vi "DevRef Data Base fg.vi"(9 "DevRef to Get":T11, 11 "Menu":T12) -> (0 "error out":errorcluster, 1 "Selected Sensor":T1, 2 "Selected Encoder":T4={"DevStatus"={"status"=FALSE, "code"=0, "source"=""}, "EncoderIndex"=enum."Invalid", "CounterIndex"=enum."Invalid", "DistancePerCount"=1.0, "Decoding Type"=enum."4x"}, 3 "Selected Solenoid":T8={"DevStatus"={"status"=FALSE, "code"=0, "source"=""}, "Solenoid Module"=enum."Solenoid Module 1", "Forward Solenoid Channel"=enum."Invalid", "Reverse Solenoid Channel"=enum."Invalid"}, 4 "autoshoot":T1, 5 "right drive encoder":T4={"DevStatus"={"status"=FALSE, "code"=0, "source"=""}, "EncoderIndex"=enum."Invalid", "CounterIndex"=enum."Invalid", "DistancePerCount"=1.0, "Decoding Type"=enum."4x"}, 6 "hotgoal":T1, 7 "left drive encoder":T4={"DevStatus"={"status"=FALSE, "code"=0, "source"=""}, "EncoderIndex"=enum."Invalid", "CounterIndex"=enum."Invalid", "DistancePerCount"=1.0, "Decoding Type"=enum."4x"}, 8 "2ball":T1)   [LabVIEW 2013]
uses:
  typedefs/fg_typedef.ctl
  typedefs/DevRef Type.ctl
  <vilib>/Rock Robotics/WPI/Solenoid/WPI_SolenoidDevRef.ctl
  <vilib>/Rock Robotics/SystemInterfaces/Typedef/FPGA_TypedefSolenoidModule.ctl
  <vilib>/Rock Robotics/WPI/Solenoid/WPI_SolenoidChannel.ctl
  <vilib>/Rock Robotics/WPI/DigitalInput/WPI_DigitalInputDevRef.ctl
  <vilib>/Rock Robotics/SystemInterfaces/DIO/FPGA_DIOChannel.ctl
  <vilib>/Rock Robotics/SystemInterfaces/Typedef/FPGA_TypedefDigitalModule.ctl
  <vilib>/Rock Robotics/WPI/Encoder/WPI_EncoderDevRef.ctl
  <vilib>/Rock Robotics/SystemInterfaces/Encoder/FPGA_EncoderIdx.ctl
  <vilib>/Rock Robotics/SystemInterfaces/Counter/FPGA_CounterCtrSystemIndex.ctl
  <vilib>/Rock Robotics/WPI/Encoder/WPI_EncoderType.ctl
panel:
  # "A Functional Global that stores refnums for \ncommonly used devices \nso as to not need to get them repeatedly"
  # "it is only set once"
  # "Option to Select Also..."
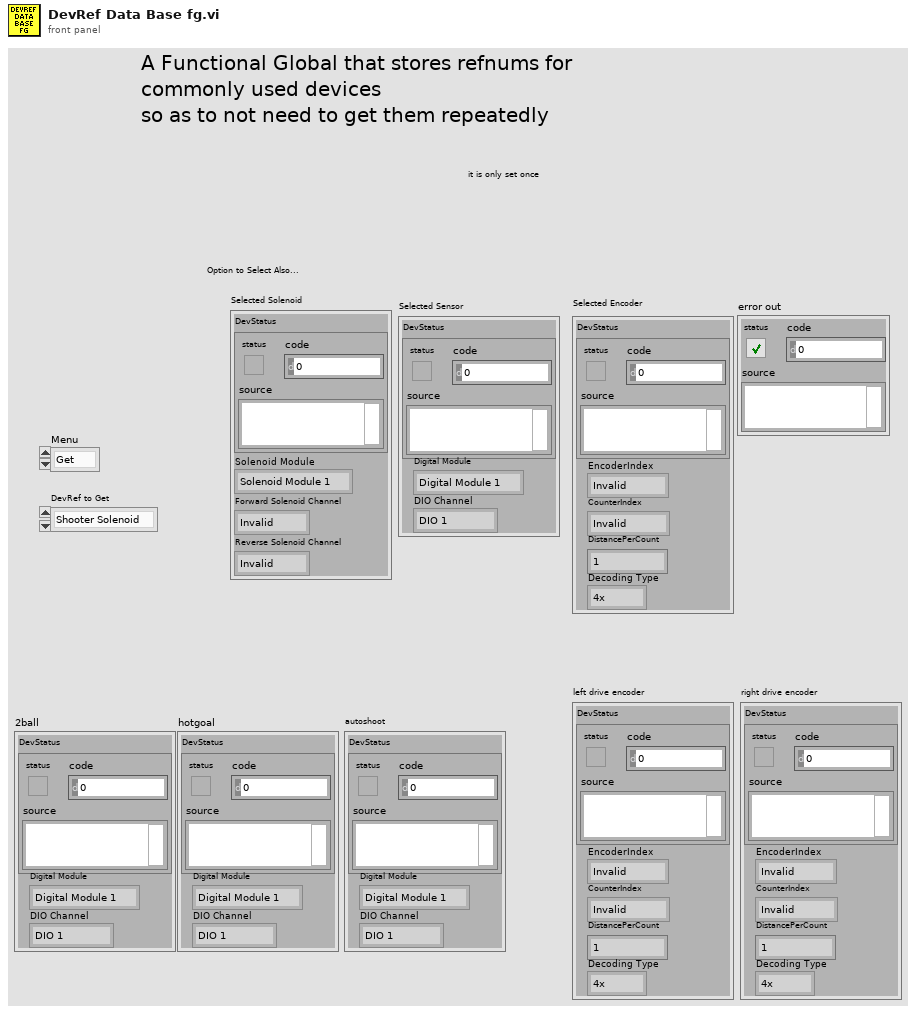
[diagram p1: front panel]
types:
  T1 = typedef "WPI_DigitalInputDevRef.ctl" = cluster{"DevStatus":errorcluster, "DIO Channel":T2, "Digital Module":T3}
  T2 = typedef "FPGA_DIOChannel.ctl" = enum8{"DIO 1", "DIO 2", "DIO 3", "DIO 4", "DIO 5", "DIO 6", "DIO 7", "DIO 8", "DIO 9", "DIO 10", "DIO 11", "DIO 12", "DIO 13", "DIO 14", "Invalid"}
  T3 = typedef "FPGA_TypedefDigitalModule.ctl" = enum16{"Digital Module 1", "Digital Module 2"}
  T4 = typedef "WPI_EncoderDevRef.ctl" = cluster{"DevStatus":errorcluster, "EncoderIndex":T5, "CounterIndex":T6, "DistancePerCount":dbl, "Decoding Type":T7}
  T5 = typedef "FPGA_EncoderIdx.ctl" = enum8{"Enc 0", "Enc 1", "Enc 2", "Enc 3", "Invalid"}
  T6 = typedef "FPGA_CounterCtrSystemIndex.ctl" = enum8{"Ctr 0", "Ctr 1", "Ctr 2", "Ctr 3", "Ctr 4", "Ctr 5", "Ctr 6", "Ctr 7", "Invalid"}
  T7 = typedef "WPI_EncoderType.ctl" = enum16{"1x", "2x", "4x"}
  T8 = typedef "WPI_SolenoidDevRef.ctl" = cluster{"DevStatus":errorcluster, "Solenoid Module":T9, "Forward Solenoid Channel":T10, "Reverse Solenoid Channel":T10}
  T9 = typedef "FPGA_TypedefSolenoidModule.ctl" = enum16{"Solenoid Module 1", "Solenoid Module 2"}
  T10 = typedef "WPI_SolenoidChannel.ctl" = enum8{"Solenoid 1", "Solenoid 2", "Solenoid 3", "Solenoid 4", "Solenoid 5", "Solenoid 6", "Solenoid 7", "Solenoid 8", "Invalid"}
  T11 = typedef "DevRef Type.ctl" = enum16{"Shooter Solenoid", "Latch Solenoid", "Right Up Sensor", "Right Down Sensor", "Hold Sensor", "Arm Encoder"}
  T12 = typedef "fg_typedef.ctl" = enum16{"Get", "Set"}
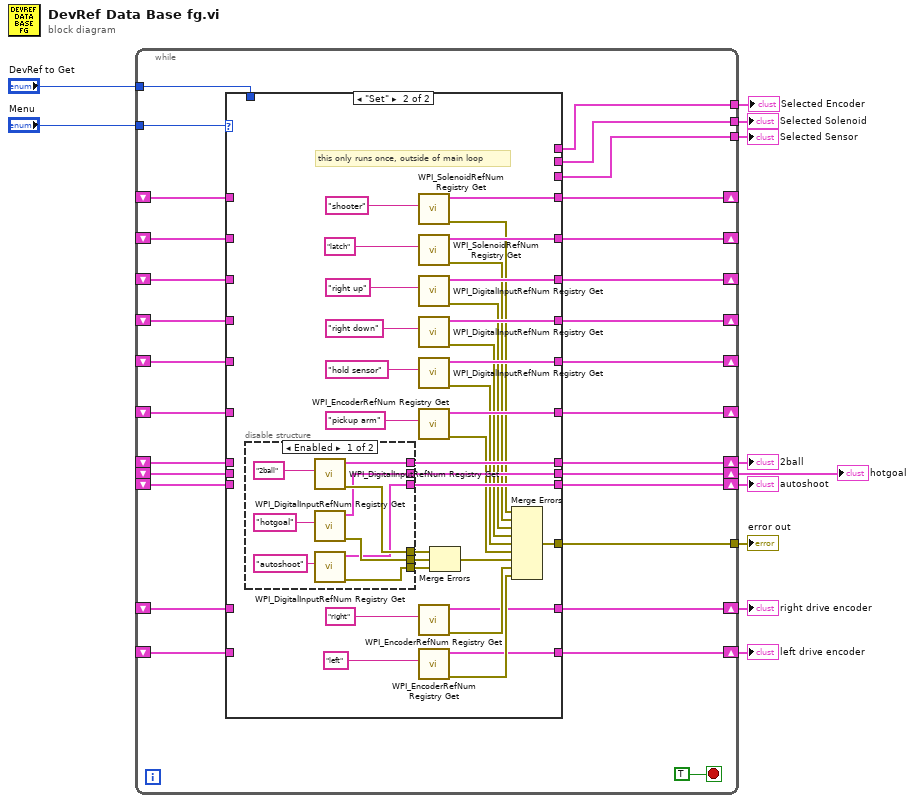
[diagram p0: block diagram]
diagram:
  n1 = while {
    shift-right: [w34] -> _
    shift-left: _ -> [w39]
    shift-right: [w33] -> _
    shift-left: _ -> [w38]
    shift-right: [w32] -> _
    shift-left: _ -> [w36]
    shift-right: [w31] -> _
    shift-left: _ -> [w35]
    tunnel: "Menu" -> [w37]
    shift-right: [w29] -> _
    shift-left: _ -> [w30]
    tunnel: "DevRef to Get" -> [w28]
    tunnel: [w27] -> w9
    tunnel: [w26] -> w8
    shift-right: [w24] -> _
    shift-left: _ -> [w25]
    tunnel: [w23] -> w7
    shift-right: [w22] -> w3
    shift-left: _ -> [w21]
    shift-right: [w20] -> w5
    shift-left: _ -> [w17]
    shift-right: [w19] -> w4
    shift-left: _ -> [w16]
    tunnel: [w18] -> w6
    shift-right: [w15] -> w2
    shift-left: _ -> [w13]
    shift-right: [w14] -> w1
    shift-left: _ -> [w12]
    stop <- TRUE stop-if-true
    n2 = case shown="\"Set\"" w37 {
      tunnel: w39 -> [w60 _]
      tunnel: w38 -> [w59 _]
      tunnel: w36 -> [w58 _]
      tunnel: w35 -> [w57 _]
      tunnel: [w49 w122] -> w34
      tunnel: [w50 w121] -> w33
      tunnel: [w51 w120] -> w32
      tunnel: [w52 w119] -> w31
      tunnel: w30 -> [w56 _]
      tunnel: [w53 w118] -> w29
      tunnel: w28 -> [w61 _]
      tunnel: [w55 _] -> w27
      tunnel: [w54 _] -> w26
      tunnel: w25 -> [w48 _]
      tunnel: [w47 w116] -> w24
      tunnel: [w46 _] -> w23
      tunnel: [w43 w115] -> w22
      tunnel: w21 -> [w43 _]
      tunnel: [w45 w104] -> w20
      tunnel: [w44 w103] -> w19
      tunnel: [_ w102] -> w18
      tunnel: w17 -> [w45 _]
      tunnel: w16 -> [w44 _]
      tunnel: [w42 w129] -> w15
      tunnel: [w41 w128] -> w14
      tunnel: w13 -> [w42 _]
      tunnel: w12 -> [w41 _]
      frame "Get", Default {
        # "always get the autobox"
        # "always get the drive encoders"
        n3 = case shown="\"Shooter Solenoid\", Default" w61 {
          tunnel: w60 -> [w63 w73 w79 w85 w91 w97]
          tunnel: w59 -> [w64 w72 w78 w84 w90 w96]
          tunnel: w58 -> [w65 w71 w77 w83 w89 w95]
          tunnel: w57 -> [w66 w70 w76 w82 w88 w94]
          tunnel: w56 -> [w67 w69 w75 w81 w87 w93]
          tunnel: [w63 w72 _ _ _ _] -> w55
          tunnel: [_ _ w77 w82 w87 _] -> w54
          tunnel: [w67 w69 w75 w81 w87 w93] -> w53
          tunnel: [w66 w70 w76 w82 w88 w94] -> w52
          tunnel: [w65 w71 w77 w83 w89 w95] -> w51
          tunnel: [w64 w72 w78 w84 w90 w96] -> w50
          tunnel: [w63 w73 w79 w85 w91 w97] -> w49
          tunnel: w48 -> [w62 w68 w74 w80 w86 w92]
          tunnel: [w62 w68 w74 w80 w86 w92] -> w47
          tunnel: [_ _ _ _ _ w92] -> w46
          frame "Shooter Solenoid", Default {
          }
          frame "Latch Solenoid" {
          }
          frame "Right Up Sensor" {
          }
          frame "Right Down Sensor" {
          }
          frame "Hold Sensor" {
          }
          frame "Arm Encoder" {
          }
        }
      }
      frame "Set" {
        # "this only runs once, outside of main loop"
        n4 = disable-structure shown="Enabled" {
          disable-tunnel: [w134 _] -> w115
          disable-tunnel: [w131 _] -> w129
          disable-tunnel: [w130 _] -> w128
          disable-tunnel: [w138 _] -> w101
          disable-tunnel: [w137 _] -> w100
          disable-tunnel: [w136 _] -> w99
          frame Enabled {
            n5 = call <vilib>:"WPI_DigitalInputRefNum Registry Get.vi"("refnum name"="2ball") -> ("error out"=w138:errorcluster, "DigitalInputDevRef"=w134:T1)  [unwired: 9 in]
            n6 = call <vilib>:"WPI_DigitalInputRefNum Registry Get.vi"("refnum name"="hotgoal") -> ("error out"=w137:errorcluster, "DigitalInputDevRef"=w131:T1)  [unwired: 9 in]
            n7 = call <vilib>:"WPI_DigitalInputRefNum Registry Get.vi"("refnum name"="autoshoot") -> ("error out"=w136:errorcluster, "DigitalInputDevRef"=w130:T1)  [unwired: 9 in]
          }
          frame Disabled {
          }
        }
        n8 = call <vilib>:"WPI_SolenoidRefNum Registry Get.vi"("refnum name"="shooter") -> ("error out"=w114:errorcluster, "SolenoidDevRef"=w122:T8)  [unwired: 9 in]
        n9 = call <vilib>:"WPI_SolenoidRefNum Registry Get.vi"("refnum name"="latch") -> ("error out"=w113:errorcluster, "SolenoidDevRef"=w121:T8)  [unwired: 9 in]
        n10 = call <vilib>:"WPI_DigitalInputRefNum Registry Get.vi"("refnum name"="right up") -> ("error out"=w112:errorcluster, "DigitalInputDevRef"=w120:T1)  [unwired: 9 in]
        n11 = call <vilib>:"WPI_DigitalInputRefNum Registry Get.vi"("refnum name"="right down") -> ("error out"=w111:errorcluster, "DigitalInputDevRef"=w119:T1)  [unwired: 9 in]
        n12 = call <vilib>:"WPI_DigitalInputRefNum Registry Get.vi"("refnum name"="hold sensor") -> ("error out"=w110:errorcluster, "DigitalInputDevRef"=w118:T1)  [unwired: 9 in]
        n13 = call <vilib>:"WPI_EncoderRefNum Registry Get.vi"("refnum name"="pickup arm") -> ("error out"=w109:errorcluster, "EncoderDevRef"=w116:T4)  [unwired: 9 in]
        n14 = call <vilib>:"WPI_EncoderRefNum Registry Get.vi"("refnum name"="right") -> ("error out"=w106:errorcluster, "EncoderDevRef"=w104:T4)  [unwired: 9 in]
        n15 = call <vilib>:"WPI_EncoderRefNum Registry Get.vi"("refnum name"="left") -> ("error out"=w105:errorcluster, "EncoderDevRef"=w103:T4)  [unwired: 9 in]
        n16 = Merge Errors(w101, w100, w99) -> (w98:errorcluster)
        n17 = Merge Errors(w114, w113, w112, w111, w110, w109, w98, w106, w105) -> (w102:errorcluster)
      }
    }
  }
  "Selected Solenoid" <- w9
  "Selected Sensor" <- w8
  "Selected Encoder" <- w7
  "error out" <- w6
  "right drive encoder" <- w5
  "left drive encoder" <- w4
  "2ball" <- w3
  "hotgoal" <- w2
  "autoshoot" <- w1
